vi "채널 8개.vi"() -> ()   [LabVIEW 2019]
uses:
  <vilib>/Math Plots/3D Math Plots/3D Scatter/3D Scatter XCtrl/3D Scatter.xctl
  <vilib>/Math Plots/3D Math Plots/3D Scatter/3D Scatter Datatype/Public/Plot Helper (Vector).vi
  <vilib>/Math Plots/3D Math Plots/3D Scatter/3D Scatter Datatype/3D Scatter Datatype.lvclass
panel:
  out "azimuth 배열 사이즈":i32
  out "sin(x)":dbl[](array[numeric])
  out "cos(x)":dbl[](array[numeric])
  out "오메가":dbl[](array[numeric])
  out "XZ":cluster{dbl[], dbl[]}(graph)
  out "YZ":cluster{dbl[], dbl[]}(graph)
  out "XY":cluster{dbl[], dbl[]}(graph)
  out "3D Scatter":refnum<class "3D Plot Datatype.lvclass">[](xcontrol)
  out "범위내의 X,Y,Z,반사율":cluster{dbl, dbl, dbl, u8}[](array[cluster])
  out "substring":string
  out "Array":string[](array[string])
  out "distance":dbl[](array[numeric])
  out "output array":u8[](array[numeric])
  in  "Boolean":bool
  out "xz":cluster{dbl[], dbl[]}(graph)
  out "yz":cluster{dbl[], dbl[]}(graph)
  out "XY Graph":cluster{dbl[], dbl[]}(graph)
  out "unsigned byte array":u8[][][](array[numeric])
  out "azimuth":dbl[](array[numeric])
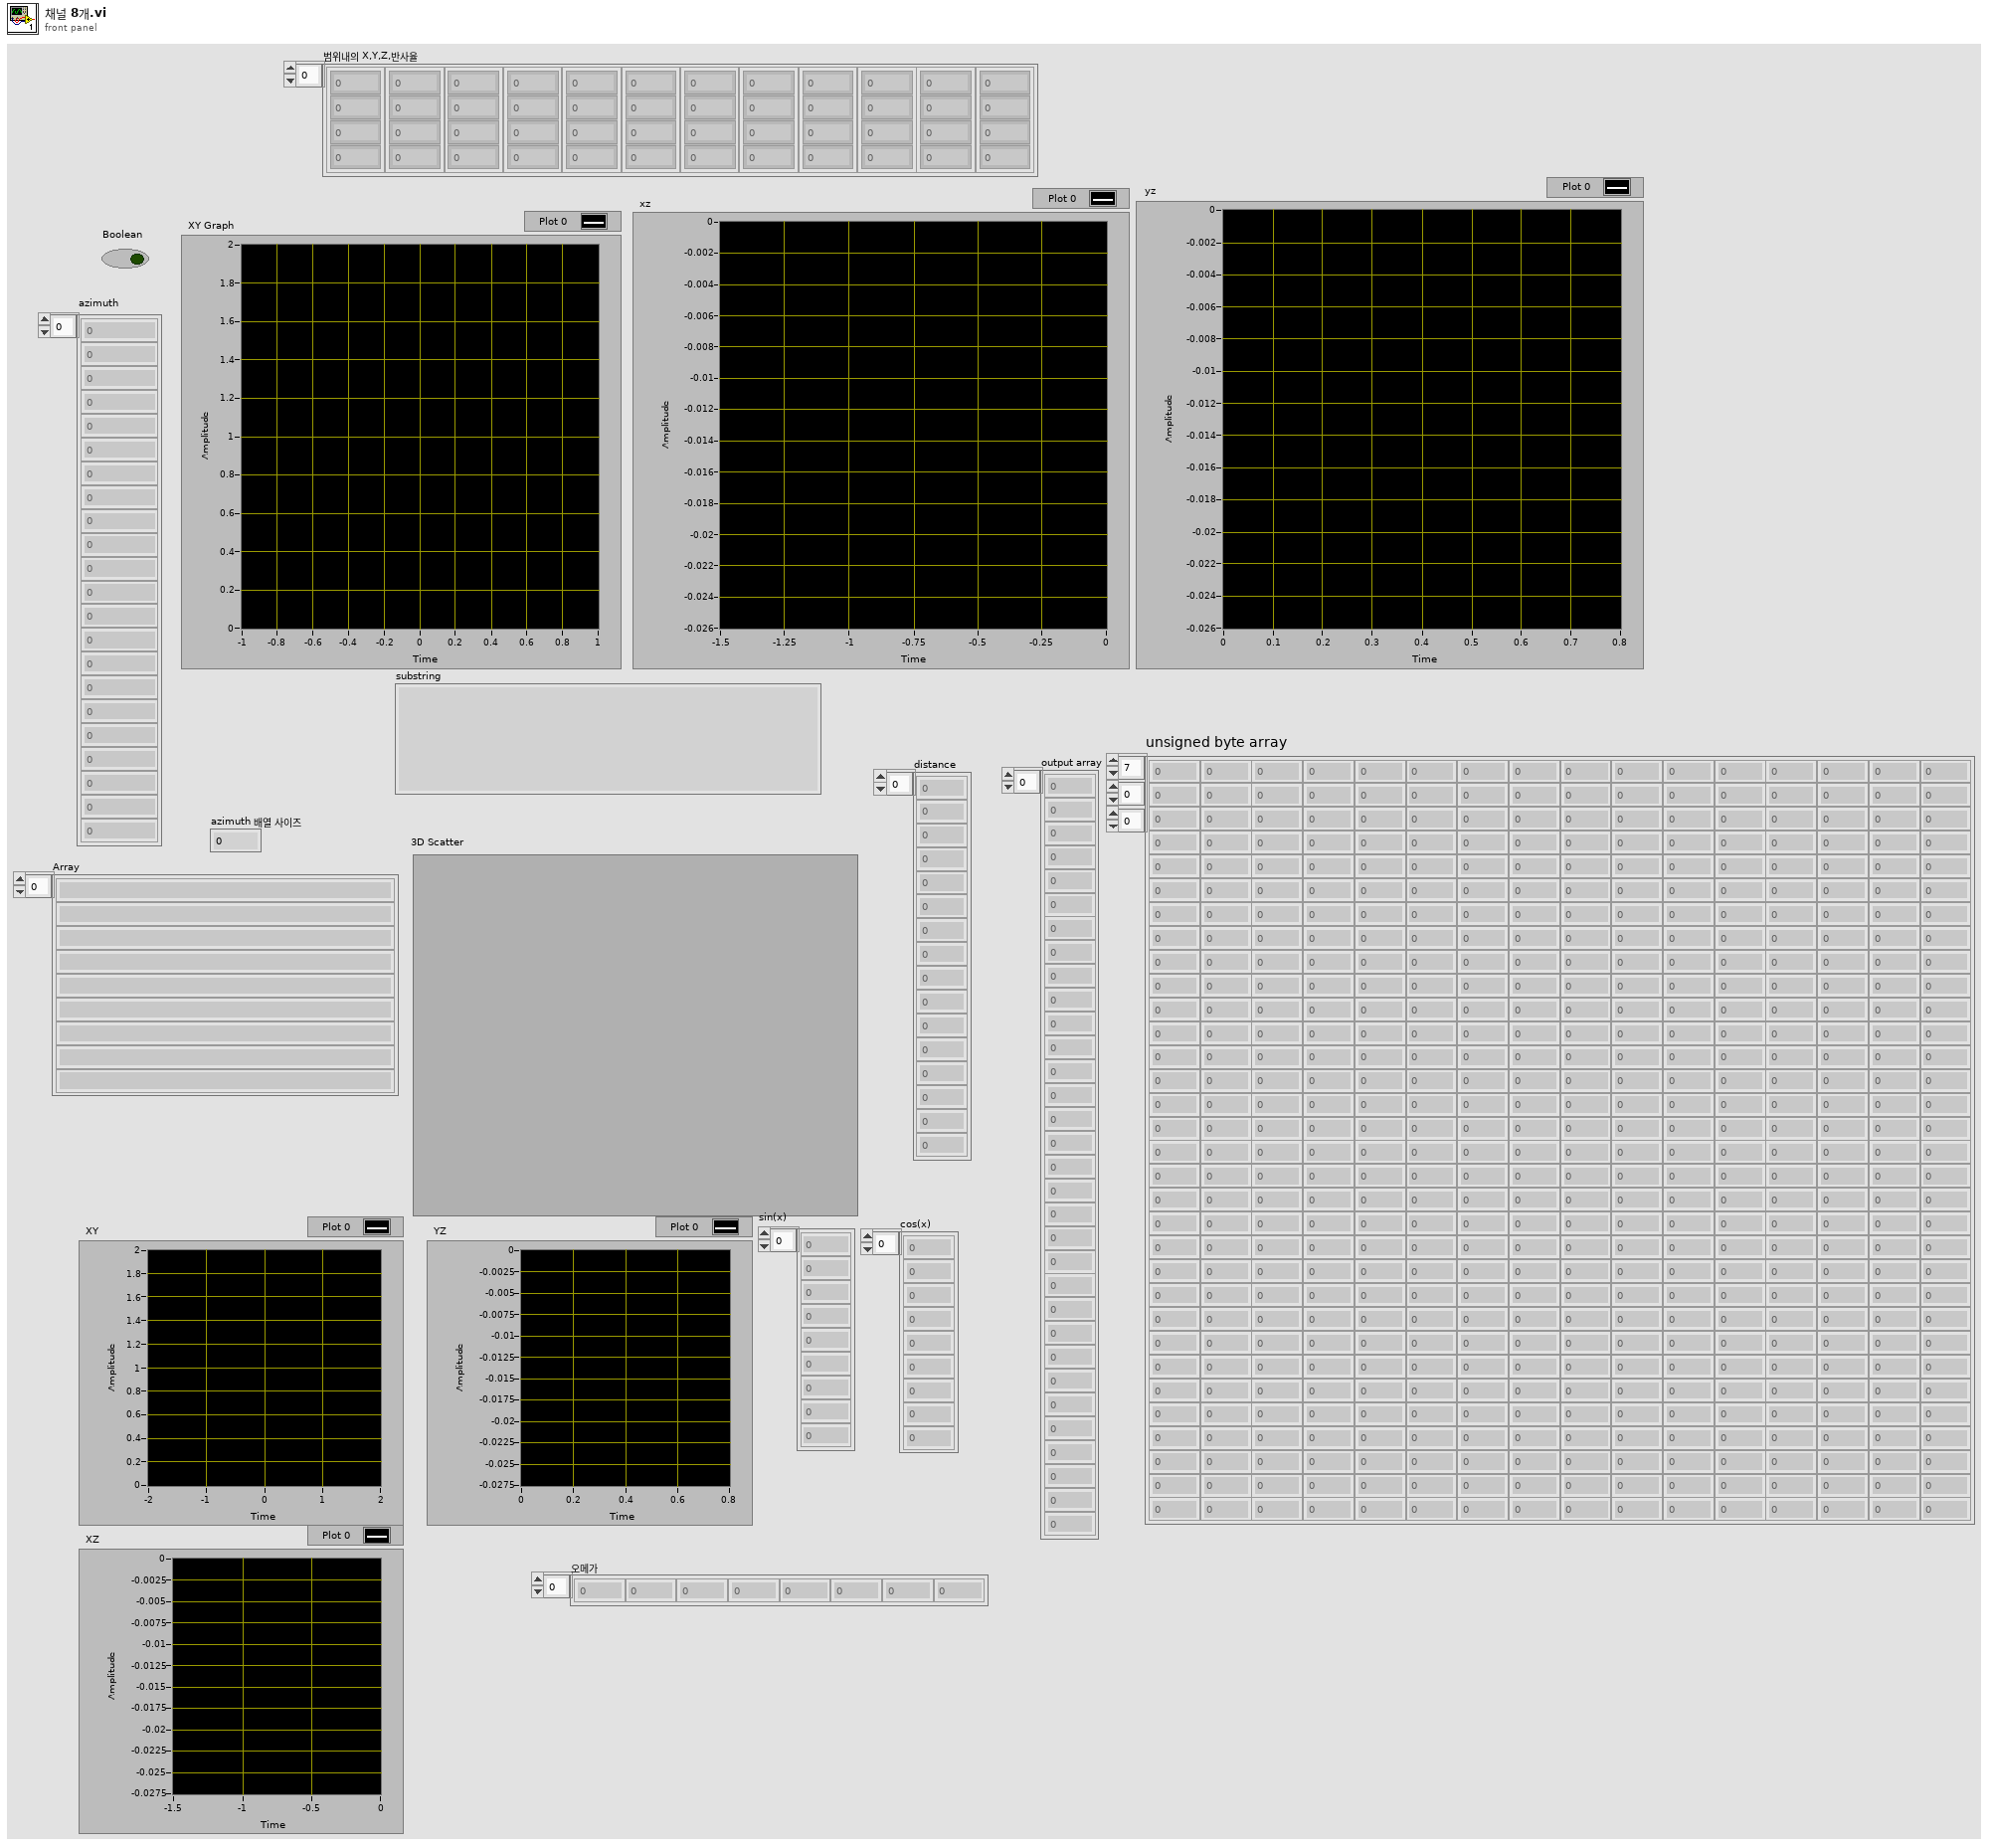
[diagram p1: front panel]
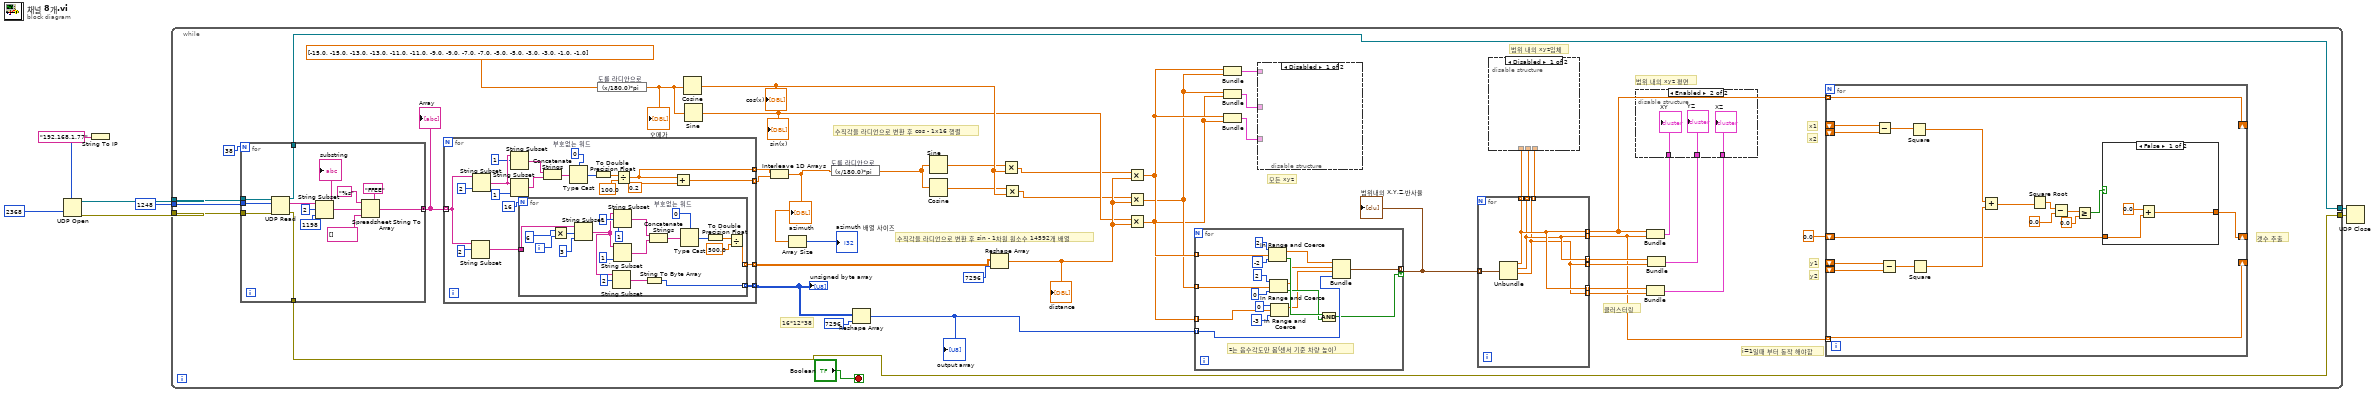
[diagram p0: block diagram]
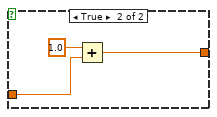
[diagram p2: hidden frame]
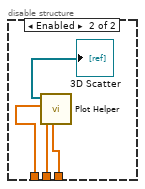
[diagram p4: hidden frame]
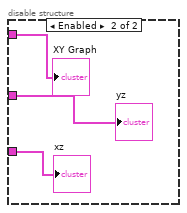
[diagram p5: hidden frame]
diagram:
  n1 = String To IP(1:"192.168.1.77") -> (0:w7:u32)
  n2 = UDP Open(7:w7, 11:2368) -> (port=w5:refnum<k16>, 0:w3:errorcluster)  [unwired: 3 in, 1 out]
  n3 = while {
    tunnel: w5 -> [w54]
    tunnel: 1248 -> [w53]
    tunnel: w3 -> [w52]
    tunnel: [w41] -> w2
    tunnel: [w12] -> w1
    stop <- "Boolean" stop-if-true
    # "갯수 추출"
    # "i=1일때 부터 동작 해야함"
    # "y2"
    # "y1"
    # "x2"
    # "x1"
    # "클러스터링"
    # "범위 내의 xyz 평면"
    # "범위 내의 xyz입체"
    # "모든 xyz"
    # "16*12*38"
    # "수직각을 라디언으로 변환 후 sin - 1차원 원소수 14592개 배열"
    # "수직각을 라디언으로 변환 후 cos - 1x16 행렬"
    n4 = for {
      N: 38 -> [_]
      tunnel: w54 -> [w163]
      tunnel: w53 -> [w162]
      tunnel: w52 -> [w161]
      tunnel: [w157] -> w41
      tunnel: [w152] -> w51 mode=concatenating
      tunnel: [w151] -> w12
      n5 = UDP Read(connection ID=w163, max size (548)=w162, 8:w161) -> (data out=w160:string, error out=w157:errorcluster, 3:w151:refnum<k16>)  [unwired: 1 in, 2 out]
      n6 = String Subset(string=w160, offset (0)=2, length (rest)=1198) -> (substring=w156:string)
      "substring" <- w156
      n7 = Spreadsheet String To Array(delimiter (Tab)="FFEE", format string="%s", spreadsheet string=w156, array type (2D Dbl)=string[] []) -> (array=w152:string[])
    }
    "Array" <- w51
    n8 = for {
      tunnel: w51 -> [w130] mode=indexing
      tunnel: [w117] -> w49 mode=indexing
      tunnel: [w116] -> w50 mode=indexing
      tunnel: [w113] -> w36 mode=indexing
      tunnel: [w112] -> w48 mode=indexing
      w111 = u16 0  # 부호없는 워드
      n9 = String Subset(string=w130, offset (0)=2) -> (substring=w114:string)  [unwired: 1 in]
      n10 = String Subset(string=w130, length (rest)=2) -> (substring=w127:string)  [unwired: 1 in]
      n11 = String Subset(string=w127, offset (0)=1) -> (substring=w124:string)  [unwired: 1 in]
      n12 = String Subset(string=w127, length (rest)=1) -> (substring=w123:string)  [unwired: 1 in]
      n13 = for {
        N: 16 -> [_]
        tunnel: w114 -> [w150]
        tunnel: [w137] -> w113 mode=indexing
        tunnel: [w133] -> w112 mode=indexing
        i -> [w149]
        w131 = u16 0  # 부호없는 워드
        n14 = Multiply(x=6, y=w149) -> (x*y=w147:i32)
        n15 = String Subset(string=w150, offset (0)=w147, length (rest)=3) -> (substring=w136:string)
        n16 = String Subset(string=w136, offset (0)=2) -> (substring=w134:string)  [unwired: 1 in]
        n17 = String Subset(string=w136, offset (0)=1, length (rest)=1 ("length (rest)")) -> (substring=w143:string)
        n18 = String Subset(string=w136, length (rest)=1) -> (substring=w142:string)  [unwired: 1 in]
        n19 = String To Byte Array(string=w134) -> (unsigned byte array=w133:u8[])
        n20 = Concatenate Strings(w143, w142) -> (w141:string)
        n21 = Type Cast(type=w131, x=w141) -> (*(type *) &x=w140:u16)
        n22 = To Double Precision Float(number=w140) -> (double precision float=w139:dbl)
        n23 = Divide(x=w139, y=500.0) -> (x/y=w137:dbl)
      }
      n24 = Concatenate Strings(w124, w123) -> (w122:string)
      n25 = Type Cast(type=w111, x=w122) -> (*(type *) &x=w121:u16)
      n26 = To Double Precision Float(number=w121) -> (double precision float=w120:dbl)
      n27 = Divide(x=w120, y=100.0) -> (x/y=w116:dbl)
      n28 = Add(x=w116, y=0.2) -> (x+y=w117:dbl)
    }
    "unsigned byte array" <- w48
    n29 = expression code="(x/180.0)*pi" "도를 라디안으로"(dbl[] [-15.0, -15.0, -13.0, -13.0, -11.0, -11.0, -9.0, -9.0, -7.0, -7.0, -5.0, -5.0, -3.0, -3.0, -1.0, -1.0]) -> (w18:dbl[])
    "오메가" <- w18
    n30 = Cosine(x=w18) -> (cos(x)=w21:dbl[])
    "cos(x)" <- w21
    n31 = Sine(x=w18) -> (sin(x)=w17:dbl[])
    "sin(x)" <- w17
    n32 = Interleave 1D Arrays(w50, w49) -> (w14:dbl[])
    "azimuth" <- w14
    n33 = Array Size(array=w14) -> (size(s)=→"azimuth 배열 사이즈":i32)
    n34 = expression code="(x/180.0)*pi" "도를 라디안으로"(w14) -> (w37:dbl[])
    n35 = Reshape Array(w48, 7296 ("차원 크기")) -> (w46:u8[])
    "output array" <- w46
    n36 = Sine(x=w37) -> (sin(x)=w20:dbl[])
    n37 = Cosine(x=w37) -> (cos(x)=w19:dbl[])
    n38 = Reshape Array(w36, 7296 ("dimension size")) -> (w35:dbl[])
    "distance" <- w35
    n39 = Multiply ("Multiply.vi")(x=w20, y=w21) -> (x*y=w16:dbl[])
    n40 = Multiply ("Multiply.vi")(x=w19, y=w21) -> (x*y=w15:dbl[])
    n41 = Multiply ("Multiply.vi")(x=w16, y=w35) -> (x*y=w40:dbl[])
    n42 = Multiply ("Multiply.vi")(x=w15, y=w35) -> (x*y=w39:dbl[])
    n43 = Multiply ("Multiply.vi")(x=w17, y=w35) -> (x*y=w38:dbl[])
    n44 = for {
      tunnel: w40 -> [w110] mode=indexing
      tunnel: w39 -> [w109] mode=indexing
      tunnel: w38 -> [w98] mode=indexing
      tunnel: w46 -> [w101] mode=indexing
      tunnel: [w100] -> w33 mode=indexing if=w99
      # "z는 음수각도만 봄(센서 기준 차량 높이)"
      n45 = In Range and Coerce(upper limit=2, x=w110, lower limit=-2) -> (coerced(x)=w103:dbl, In Range?=w105:bool)
      n46 = In Range and Coerce(upper limit=2, x=w109, lower limit=0) -> (coerced(x)=w102:dbl, In Range?=w104:bool)
      n47 = In Range and Coerce(upper limit=0, x=w98, lower limit=-3) -> (coerced(x)=w96:dbl)  [unwired: 1 out]
      n48 = Compound Arithmetic op=AND(w105, w104) -> (w99:bool)
      n49 = Bundle(w103, w102, w96, w101) -> (w100:cluster{dbl, dbl, dbl, u8})  [unwired: 1 in]
    }
    "범위내의 X,Y,Z,반사율" <- w33
    n50 = Bundle(w40, w39) -> (w45:cluster{dbl[], dbl[]})  [unwired: 1 in]
    n51 = Bundle(w39, w38) -> (w44:cluster{dbl[], dbl[]})  [unwired: 1 in]
    n52 = Bundle(w40, w38) -> (w43:cluster{dbl[], dbl[]})  [unwired: 1 in]
    n53 = disable-structure shown="Disabled" {
      disable-tunnel: w45 -> [_ w93]
      disable-tunnel: w44 -> [_ w92]
      disable-tunnel: w43 -> [_ w91]
      frame Disabled {
      }
      frame Enabled {
        "XY Graph" <- w93
        "yz" <- w92
        "xz" <- w91
      }
    }
    n54 = for {
      tunnel: w33 -> [w90] mode=indexing
      tunnel: [w89] -> w11 mode=indexing
      tunnel: [w88] -> w10 mode=indexing
      tunnel: [w87] -> w32 mode=indexing
      tunnel: [w88] -> w31 mode=indexing
      tunnel: [w89] -> w30 mode=indexing
      tunnel: [w87] -> w29 mode=indexing
      tunnel: [w89] -> w28 mode=indexing
      tunnel: [w88] -> w27 mode=indexing
      tunnel: [w87] -> w26 mode=indexing
      n55 = Unbundle(w90) -> (w89:dbl, w88:dbl, w87:dbl)  [unwired: 1 out]
    }
    n56 = disable-structure shown="Disabled" {
      disable-tunnel: w28 -> [_ w85]
      disable-tunnel: w27 -> [_ w84]
      disable-tunnel: w26 -> [_ w83]
      frame Disabled {
      }
      frame Enabled {
        n57 = call-poly <vilib>:"Plot Helper.vi"("z vector"=w83, "y vector"=w84, "x vector"=w85) -> ("3D Plot lvclass Array out"=→"3D Scatter":refnum<class "3D Plot Datatype.lvclass">[])  [unwired: 3 in, 5 out]
      }
    }
    n58 = Bundle(w11, w10) -> (w25:cluster{dbl[], dbl[]})  [unwired: 1 in]
    n59 = Bundle(w30, w29) -> (w23:cluster{dbl[], dbl[]})  [unwired: 1 in]
    n60 = Bundle(w31, w32) -> (w24:cluster{dbl[], dbl[]})  [unwired: 1 in]
    n61 = disable-structure shown="Enabled" {
      disable-tunnel: w25 -> [_ w80]
      disable-tunnel: w24 -> [_ w82]
      disable-tunnel: w23 -> [_ w81]
      frame Disabled {
      }
      frame Enabled {
        "XY" <- w80
        "YZ" <- w82
        "XZ" <- w81
      }
    }
    n62 = for {
      tunnel: w11 -> [w73] mode=indexing
      tunnel: w10 -> [w72] mode=indexing
      shift-right: [w73] -> _
      shift-left: _ -> [w71]
      shift-left: _ -> [w70]
      shift-right: [w72] -> _
      shift-left: _ -> [w67]
      shift-left: _ -> [w66]
      shift-right: [w56] -> _
      shift-left: 0.0 -> [w57]
      n63 = Subtract(x=w71, y=w70) -> (x-y=w69:dbl)
      n64 = Subtract(x=w67, y=w66) -> (x-y=w68:dbl)
      n65 = Square(x=w69) -> (x^2=w65:dbl)
      n66 = Square(x=w68) -> (x^2=w64:dbl)
      n67 = Add(x=w65, y=w64) -> (x+y=w63:dbl)
      n68 = Square Root(x=w63) -> (sqrt(x)=w62:dbl)
      n69 = Subtract(x=w62, y=0.0) -> (x-y=w60:dbl)
      n70 = Greater Or Equal?(x=w60, y=0.0) -> (x >= y?=w58:bool)
      n71 = case shown="False" w58 {
        tunnel: w57 -> [w74 w78]
        tunnel: [w75 w77] -> w56
        frame False {
          n72 = Add(x=0.0, y=w74) -> (x+y=w75:dbl)
        }
        frame True {
          n73 = Add(x=1.0, y=w78) -> (x+y=w77:dbl)
        }
      }
    }
  }
  n74 = UDP Close(connection ID=w1, 8:w2) -> ()  [unwired: 2 out]
